vi "AlliGator Decode Python Plugin Output Section.vi"(8 "error in (no error)":errorcluster, 9 "Source":string, 11 "Input String":string) -> (0 "error out":errorcluster, 2 "Function Outputs":T1[](array[typedef]), 3 "Output String":string)   [LabVIEW 2021, in "AlliGator Python Plugins.lvlib"]
doc: "Looks for Python Plugin Header and Footer and returns:\n\n- String before Header\n- <B>Output Type</B>\n- <B>Output Destination</B>\n\n<B>String before Header</B>: isf the section is not found (no header or no footer), the input string is passed unchanged.\n\nIf the section is found, the part that preceded that section is returned,"
uses:
  AlliGator Python Plugins.lvlib
  AlliGator Python Function Output Definition.ctl
  Strings/Strings.lvlib
panel:
  # "see the AlliGator License on the block diagram (Ctrl+E or Window:Show Block Diagram)"
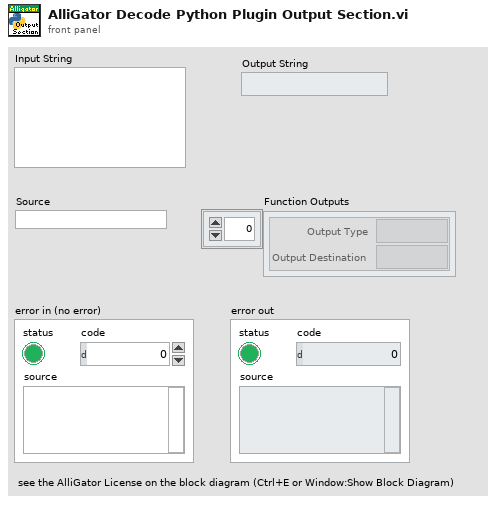
[diagram p1: front panel]
types:
  T1 = typedef "AlliGator Python Plugins.lvlib/AlliGator Python Function Output Definition.ctl" = cluster{"Output Type":string, "Output Destination":string}
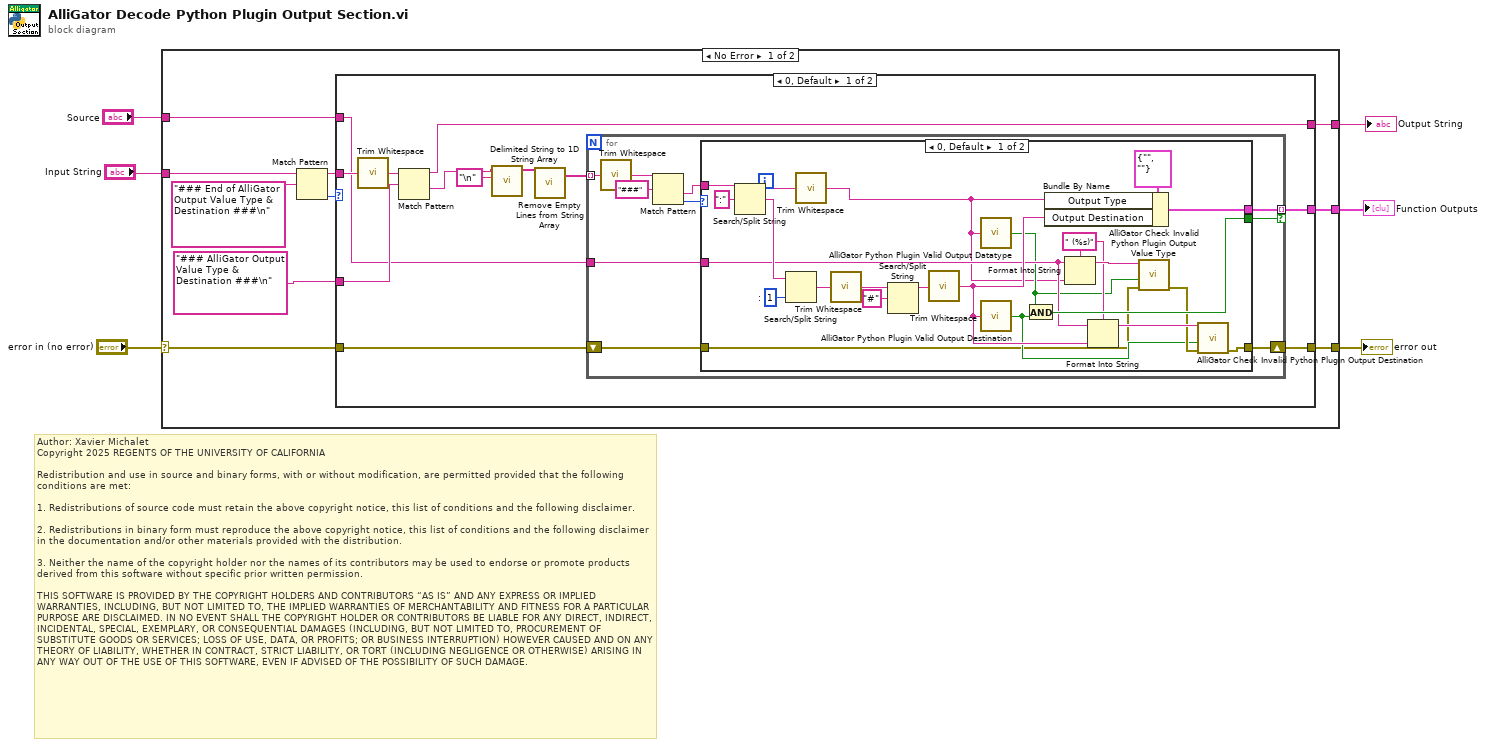
[diagram p0: block diagram]
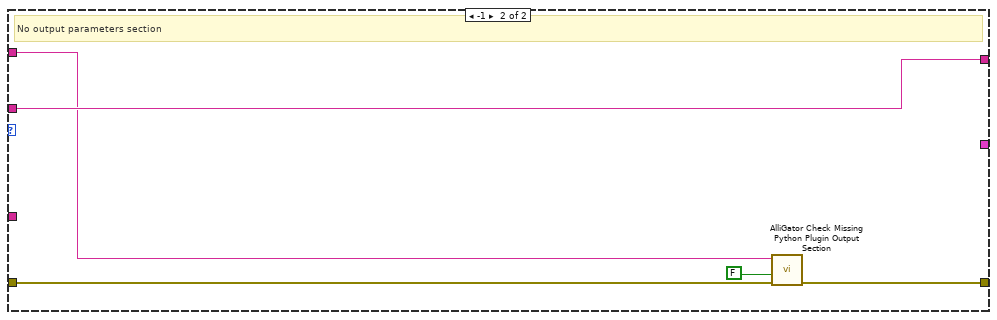
[diagram p3: hidden frame]
diagram:
  # "Author: Xavier Michalet\nCopyright 2025 REGENTS OF THE UNIVERSITY OF CALIFORNIA\n\nRedistribution and use in source and binary forms, with or without modification, are permitted provided that the following conditions are met:\n\n1. Redistributions of source code must retain the above copyright notice, this list of conditions and the following disclaimer.\n\n2. Redistributions in binary form must reproduce the above copyright notice, this list of conditions and the following disclaimer in the documentation and/or other materials provided with the distribution.\n\n3. Neither the name of the copyright holder nor the names of its contributors may be used to endorse or promote products derived from this software without specific prior written permission.\n\nTHIS SOFTWARE IS PROVIDED BY THE COPYRIGHT HOLDERS AND CONTRIBUTORS “AS IS” AND ANY EXPRESS OR IMPLIED WARRANTIES, INCLUDING, BUT NOT LIMITED TO, THE IMPLIED WARRANTIES OF MERCHANTABILITY AND FITNESS FOR A PARTICULAR PURPOSE ARE DISCLAIMED. IN NO EVENT SHALL THE COPYRIGHT HOLDER OR CONTRIBUTORS BE LIABLE FOR ANY DIRECT, INDIRECT, INCIDENTAL, SPECIAL, EXEMPLARY, OR CONSEQUENTIAL DAMAGES (INCLUDING, BUT NOT LIMITED TO, PROCUREMENT OF SUBSTITUTE GOODS OR SERVICES; LOSS OF USE, DATA, OR PROFITS; OR BUSINESS INTERRUPTION) HOWEVER CAUSED AND ON ANY THEORY OF LIABILITY, WHETHER IN CONTRACT, STRICT LIABILITY, OR TORT (INCLUDING NEGLIGENCE OR OTHERWISE) ARISING IN ANY WAY OUT OF THE USE OF THIS SOFTWARE, EVEN IF ADVISED OF THE POSSIBILITY OF SUCH DAMAGE."
  n1 = case shown="No Error" "error in (no error)" {
    selector: "error in (no error)" -> [w16 w69]
    tunnel: [w15 w69] -> w5
    tunnel: "Input String" -> [w13 w68]
    tunnel: [w11 w68] -> w3
    tunnel: "Source" -> [w8 _]
    tunnel: [w7 _] -> w1
    frame No Error {
      n2 = Match Pattern(string=w13, regular expression="### End of AlliGator Output Value Type & Destination ###\n") -> (before substring=w14:string, offset past match=w12:i32)  [unwired: 1 in, 2 out]
      n3 = case shown="0, Default" w12 {
        tunnel: w14 -> [w26 w65]
        tunnel: "### AlliGator Output Value Type & Destination ###\n" ("regular expression") -> [w24 _]
        tunnel: [w18 w66] -> w15
        tunnel: w16 -> [w19 w67]
        tunnel: [w21 w65] -> w11
        tunnel: w8 -> [w20 w63]
        tunnel: [w17 _] -> w7
        frame 0, Default {
          n4 = call <vilib>:"Trim Whitespace.vi"("string"=w26) -> ("trimmed string"=w22:string)  [unwired: 1 in]
          n5 = Match Pattern(string=w22, regular expression=w24) -> (before substring=w21:string, after substring=w23:string)  [unwired: 1 in, 2 out]
          n6 = call <vilib>:"Delimited String to 1D String Array.vi"("delimiter"="\n", "delimited string"=w23) -> ("string array"=w28:string[])  [unwired: 9 in]
          n7 = call "Remove Empty Lines from String Array.vi"("string array in"=w28) -> ("string array out"=w25:string[])
          n8 = for {
            tunnel: w25 -> [w38] mode=indexing
            tunnel: [w34] -> w17 mode=indexing if=w33
            tunnel: w20 -> [w32]
            shift-right: [w31] -> w18
            shift-left: w19 -> [w30]
            n9 = call <vilib>:"Trim Whitespace.vi"("string"=w38) -> ("trimmed string"=w36:string)  [unwired: 1 in]
            n10 = Match Pattern(string=w36, regular expression="###") -> (after substring=w29:string, offset past match=w35:i32)  [unwired: 1 in, 2 out]
            n11 = case shown="0, Default" w35 {
              tunnel: w29 -> [w53 _]
              tunnel: [w51 _] -> w34
              tunnel: [w50 _] -> w33
              tunnel: w32 -> [w45 _]
              tunnel: [w41 w62] -> w31
              tunnel: w30 -> [w40 w62]
              frame 0, Default {
                w47 = " (%s)" ("format string")
                w59 = 1  # :
                n12 = Search/Split String(string=w53, search string/char (-)=":") -> (substring before match=w55:string, match + rest of string=w60:string)  [unwired: 1 in, 1 out]
                n13 = Search/Split String(string=w60, offset (0)=w59) -> (match + rest of string=w57:string)  [unwired: 1 in, 2 out]
                n14 = call <vilib>:"Trim Whitespace.vi"("string"=w55) -> ("trimmed string"=w39:string)  [unwired: 1 in]
                n15 = call <vilib>:"Trim Whitespace.vi"("string"=w57) -> ("trimmed string"=w54:string)  [unwired: 1 in]
                n16 = Search/Split String(string=w54, search string/char (-)="#") -> (substring before match=w56:string)  [unwired: 1 in, 2 out]
                n17 = call <vilib>:"Trim Whitespace.vi"("string"=w56) -> ("trimmed string"=w46:string)  [unwired: 1 in]
                n18 = call "AlliGator Python Plugin Valid Output Datatype.vi"("Output Datatype"=w39) -> ("Valid Datatype?"=w43:bool)  [unwired: 8 in]
                n19 = call "AlliGator Python Plugin Valid Output Destination.vi"("Output Destination"=w46) -> ("Valid Destination?"=w42:bool)  [unwired: 8 in]
                n20 = And(x=w43, y=w42) -> (x .and. y?=w50:bool)
                n21 = Bundle By Name(cluster=T1 {"Output Type"="", "Output Destination"=""} ("Python Function Output Definition"), "Output Type"=w39, "Output Destination"=w46) -> (w51:T1)
                n22 = Format Into String(format string=w47, initial string=w45, w39) -> (resulting string=w49:string)  [unwired: 1 in, 1 out]
                n23 = Format Into String(format string=w47, initial string=w45, w46) -> (resulting string=w48:string)  [unwired: 1 in, 1 out]
                n24 = call "AlliGator Check Invalid Python Plugin Output Value Type.vi"("error in (no error)"=w40, "Valid Output Value Type?"=w43, "Source"=w49) -> ("error out"=w44:errorcluster)  [unwired: 8 in]
                n25 = call "AlliGator Check Invalid Python Plugin Output Destination.vi"("error in (no error)"=w44, "Valid Destination?"=w42, "Source"=w48) -> ("error out"=w41:errorcluster)  [unwired: 8 in]
              }
              frame -1 {
              }
            }
          }
        }
        frame -1 {
          # "No output parameters section"
          n26 = call "AlliGator Check Missing Python Plugin Output Section.vi"("error in (no error)"=w67, "Output Section Found"=FALSE, "Source"=w63) -> ("error out"=w66:errorcluster)  [unwired: 8 in]
        }
      }
    }
    frame Error {
    }
  }
  "error out" <- w5
  "Output String" <- w3
  "Function Outputs" <- w1
